vi "JogX.vi"(8 "error in":errorcluster, 9 "connection refnum in":refnum<k5>, 10 "Speed (units/s)":dbl min=0.0 max=1500.0, 11 "Units":enum16{"mm", "µm"}(ring)) -> (0 "error out":errorcluster, 1 "connection refnum out":refnum<k5>)   [LabVIEW 2023]
doc: "Move in the X direction until commanded to stop\n\nWhen calling this VI from another function you must handle the stop motion action. This will not stop on its own"
uses:
  GlobalVarsNetwork.vi
panel:
  in  "Stop Button":bool
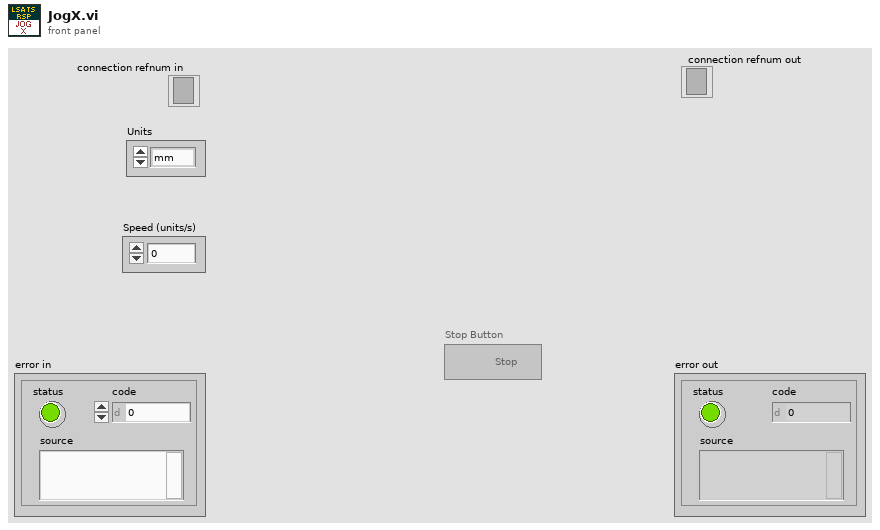
[diagram p1: front panel]
types:
  T1 = cluster{"XY_IP_ADDRESS":string, "Z_IP_ADDRESS":string, "Port":u16, "connection refnum x,y":refnum<k5>, "connection refnum z":refnum<k5>}
  T2 = enum8{"Enabled", "Disabled", "Disabled and Grayed Out"}
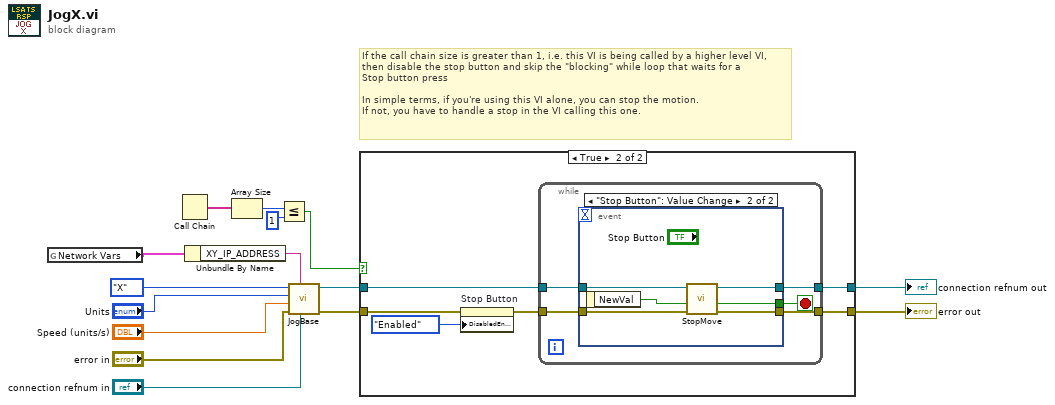
[diagram p0: block diagram]
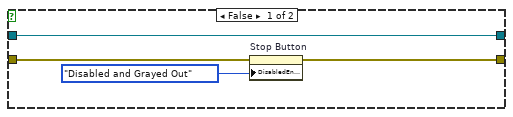
[diagram p2: hidden frame]
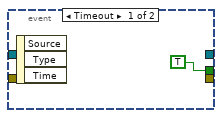
[diagram p3: hidden frame]
diagram:
  # "If the call chain size is greater than 1, i.e. this VI is being called by a higher level VI,\nthen disable the stop button and skip the \"blocking\" while loop that waits for a \nStop button press\n\nIn simple terms, if you're using this VI alone, you can stop the motion.\nIf not, you have to handle a stop in the VI calling this one."
  n1 = global read "GlobalVarsNetwork.vi" "Network Vars"() -> (w10:T1)
  n2 = Call Chain() -> (call chain=w9:string[])
  n3 = Unbundle By Name(w10) -> ("XY_IP_ADDRESS"=w11:string)
  n4 = Array Size(array=w9) -> (size(s)=w7:i32)
  n5 = Less Or Equal?(x=w7, y=1) -> (x <= y?=w6:bool)
  n6 = call "JogBase.vi"("connection refnum in"="connection refnum in", "IP Address"=w11, "error in"="error in", "Speed"="Speed (units/s)", "Units"="Units", "Axis"=enum16{"Z", "Y", "X"}."X") -> ("error out"=w5:errorcluster, "connection refnum out"=w2:refnum<k5>)  [unwired: 2 in]
  n7 = case shown="True" w6 {
    tunnel: w5 -> [w19 w24]
    tunnel: [w18 w25] -> w4
    tunnel: w2 -> [w16 w21]
    tunnel: [w16 w20] -> w1
    frame False {
      n8 = property on="Stop Button" class="Bool"(error in=w19, "DisabledEnum"=T2."Disabled and Grayed Out" ("Disabled")) -> (error out=w18:errorcluster)  [unwired: 1 in, 1 out]
    }
    frame True {
      n9 = property on="Stop Button" class="Bool"(error in=w24, "DisabledEnum"=T2."Enabled" ("Disabled")) -> (error out=w23:errorcluster)  [unwired: 1 in, 1 out]
      n10 = while {
        tunnel: w23 -> [w30]
        tunnel: [w29] -> w25
        tunnel: w21 -> [w27]
        tunnel: [w26] -> w20
        stop <- w28 stop-if-true
        n11 = event shown="[1] \"Stop Button\": Value Change" {
          selector: _ -> [_ _]
          dyn-events: _ -> [_ _]
          timeout: _ -> [_ _]
          tunnel: w30 -> [_ w37]
          tunnel: [_ w36] -> w29
          tunnel: [TRUE w35] -> w28
          tunnel: w27 -> [_ w33]
          tunnel: [_ w32] -> w26
          event Timeout {
            n12 = event-data() -> ()  [unwired: 1 in, 3 out]
          }
          event "Stop Button": Value Change {
            n13 = event-data() -> ("NewVal"=w34:bool)  [unwired: 1 in]
            n14 = call "StopMove.vi"("error in"=w37, "Stop?"=w34, "connection refnum in, xy"=w33) -> ("error out"=w36:errorcluster, "Stop?"=w35:bool, "connection refnum out xy"=w32:refnum<k5>)  [unwired: 1 in, 1 out]
          }
        }
      }
    }
  }
  "error out" <- w4
  "connection refnum out" <- w1
